vi "Build.vi"(6 "Assembly Type":string, 8 "Position":i32, 9 "XYZTheta":dbl[](array[numeric]), 10 "text file":dbl[][](array[numeric]), 11 "Sensor Dispense in":refnum<class "Sensor Dispense.lvclass">) -> (3 "Sensor Dispense out":refnum<class "Sensor Dispense.lvclass">)   [LabVIEW 2021, in "Sensor Dispense.lvclass"]
uses:
  Projects/Sensor Dispense.lvclass
  C:/Users/User/Documents/Jessica_Code/Jessica_code_08062024/Gantry-CMU/UCSB-Gantry-HEP-main/Classes/Routine/Dispense/Dispense.lvclass
  Projects/Sensor Dispense.lvclass/Sensor Dispense.ctl
  <vilib>/Analysis/coordinate.llb/2D Cartesian Coordinate Rotation (Scalar).vi
  <vilib>/Analysis/NI_AALPro.lvlib
panel:
  out "CW/CCW":dbl[](array[numeric])
  out "CW/CCW":dbl[](array[numeric])
  out "endpoints 2":dbl[][](array[numeric])
  out "endpoints":dbl[][](array[numeric])
  out "data":T1(array[cluster])
  out "cell count":dbl[](array[numeric])
  out "centers":dbl[][](array[numeric])
  # "[x1,y1,x2,y2]"
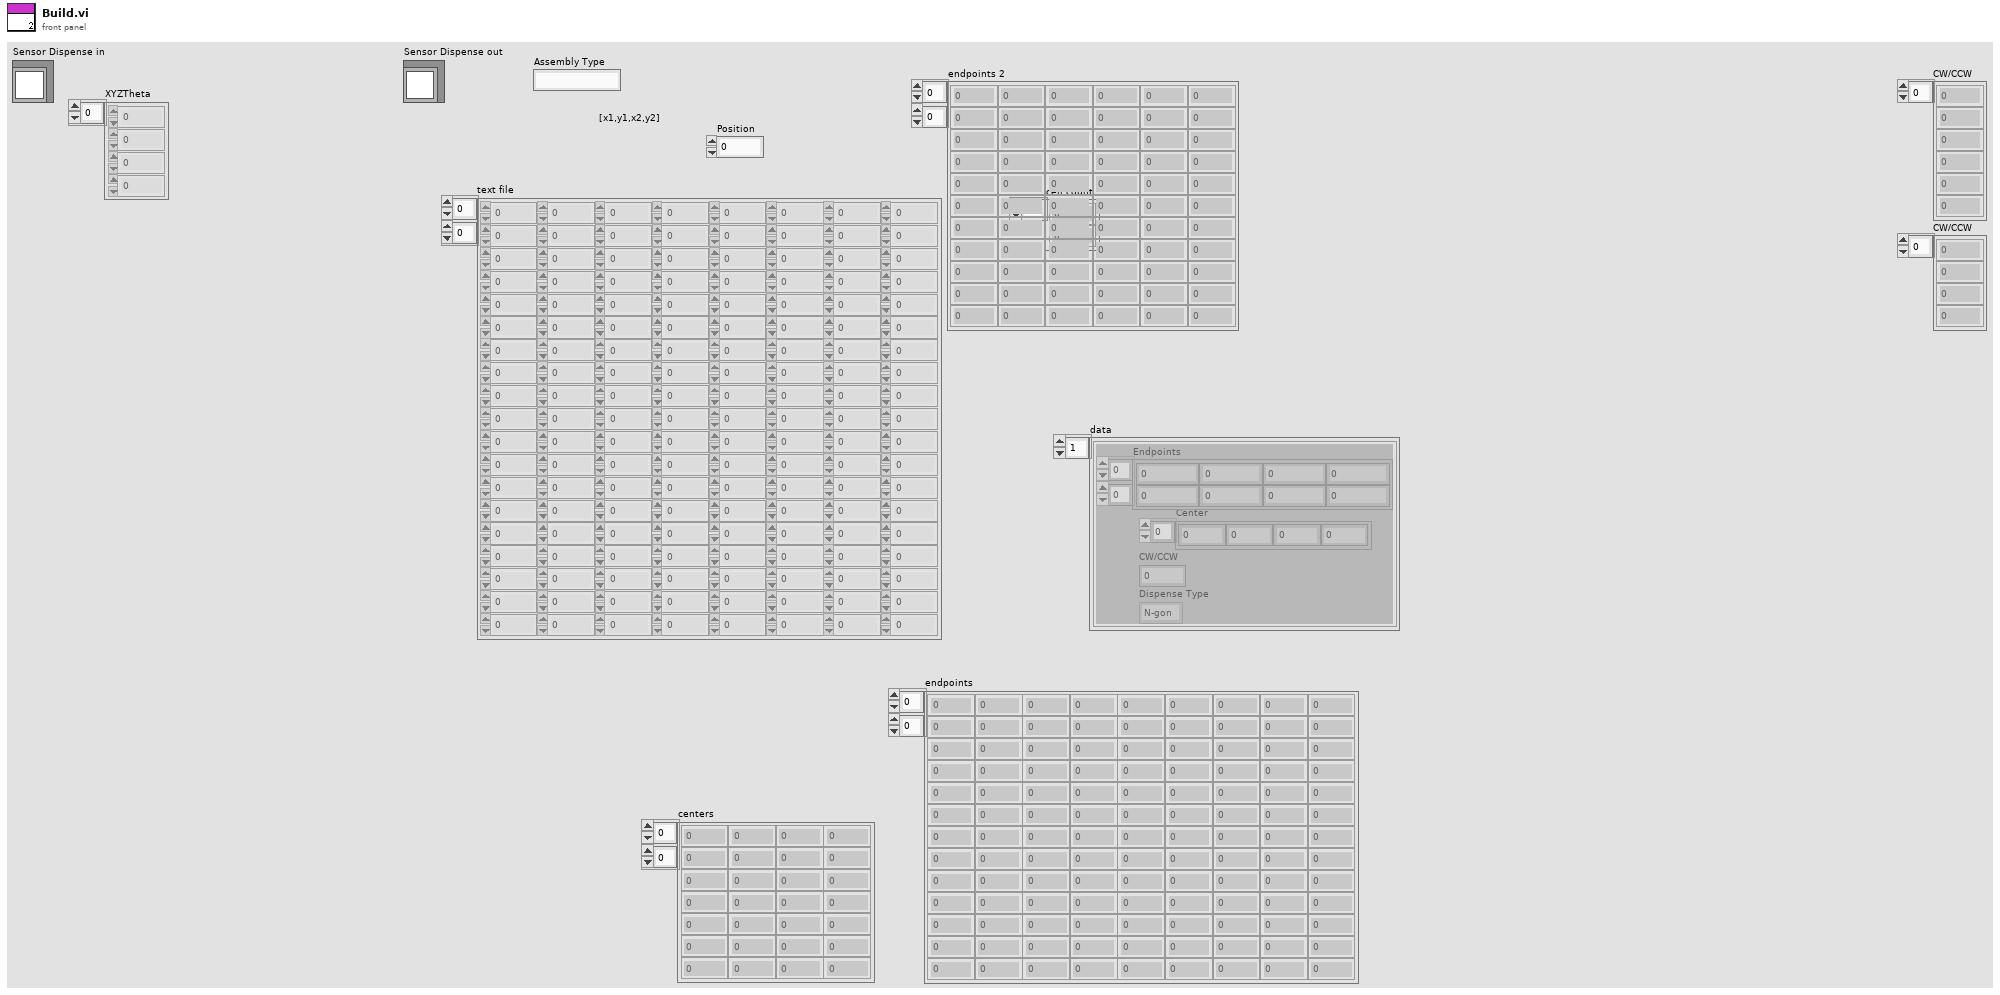
[diagram p1: front panel]
types:
  T1 = cluster{"Endpoints":dbl[][], "Center":dbl[], "CW/CCW":dbl, "Dispense Type":enum16{"N-gon", "Square", "Arc", "Dot", "Line", "Circle"}}[]
  T2 = enum16{"N-gon", "Square", "Arc", "Dot", "Line", "Circle"}
  T3 = cluster{"Endpoints":dbl[][], "Center":dbl[], "CW/CCW":dbl, "Dispense Type":enum16{"N-gon", "Square", "Arc", "Dot", "Line", "Circle"}}
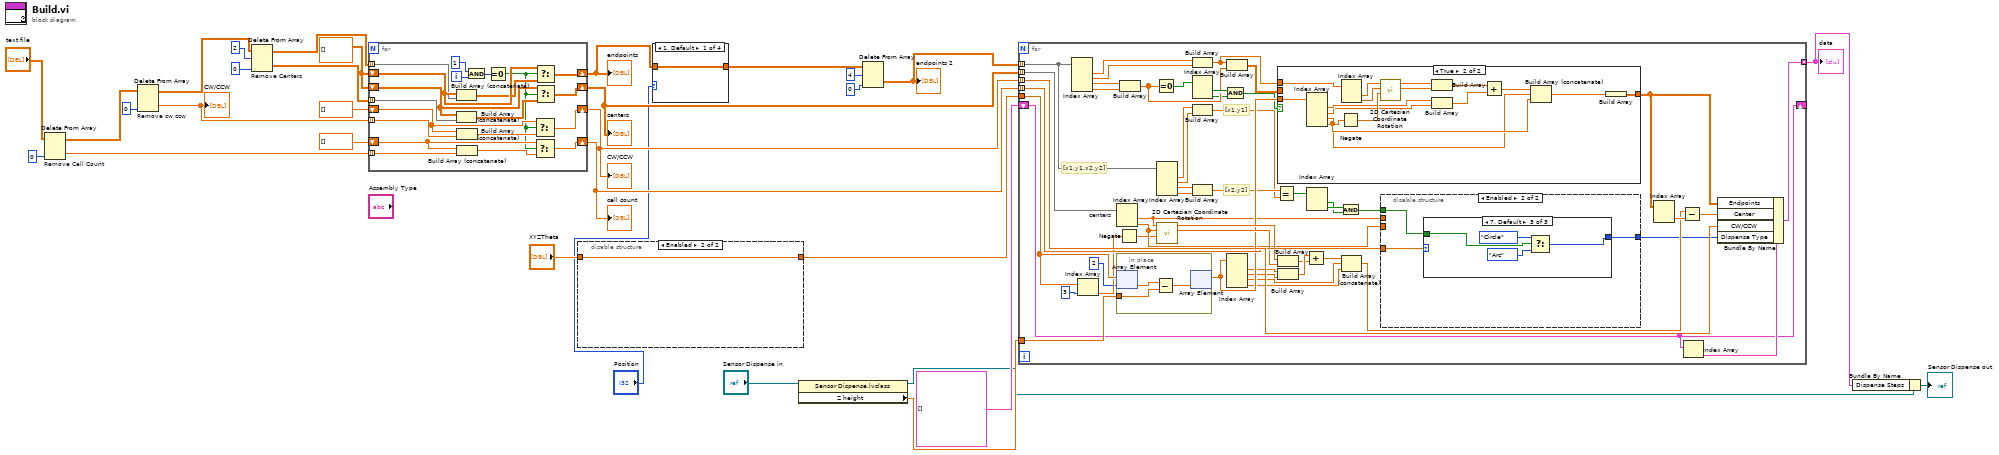
[diagram p0: block diagram]
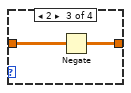
[diagram p3: hidden frame]
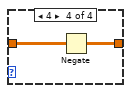
[diagram p4: hidden frame]
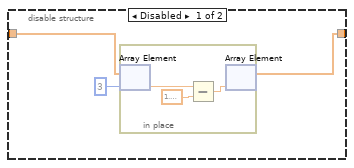
[diagram p5: hidden frame]
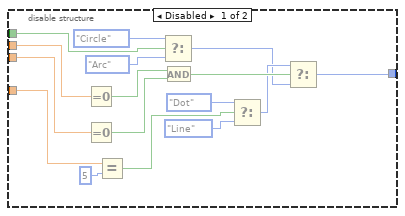
[diagram p6: hidden frame]
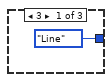
[diagram p7: hidden frame]
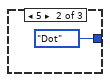
[diagram p8: hidden frame]
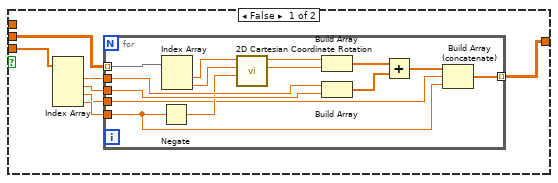
[diagram p9: hidden frame]
diagram:
  w28 = dbl[][] []
  n1 = Delete From Array "Remove Cell Count"(array="text file", index (col)=0) -> (deleted portion=w22:dbl[], array with subset deleted=w24:dbl[][])  [unwired: 2 in]
  n2 = Delete From Array "Remove cw ccw"(array=w24, index (col)=0 ("disabled index (col)")) -> (deleted portion=w5:dbl[], array with subset deleted=w21:dbl[][])  [unwired: 2 in]
  "CW/CCW" <- w5
  n3 = Delete From Array "Remove Centers"(array=w21, length=2, index (col)=0) -> (deleted portion=w17:dbl[][], array with subset deleted=w18:dbl[][])  [unwired: 1 in]
  n4 = for {
    tunnel: w18 -> [w47] mode=indexing
    shift-right: [w45] -> w1
    shift-left: w28 -> [w48]
    tunnel: w17 -> [w44] mode=indexing
    shift-right: [w41] -> w29
    shift-left: w28 -> [w42]
    tunnel: w22 -> [w40] mode=indexing
    shift-right: [w37] -> w26
    shift-left: dbl[] [] -> [w39]
    shift-right: [w32] -> w4
    shift-left: dbl[] [] -> [w35]
    tunnel: w5 -> [w36] mode=indexing
    i -> [w50]
    n5 = Build Array (concatenate)(w48, w47) -> (w46:dbl[][])
    n6 = Build Array (concatenate)(w42, w44) -> (w43:dbl[][])
    n7 = Build Array (concatenate)(w35, w36) -> (w34:dbl[])
    n8 = Build Array (concatenate)(w39, w40) -> (w38:dbl[])
    n9 = And(x=1, y=w50) -> (x .and. y?=w49:i32)
    n10 = Equal To 0?(x=w49) -> (x = 0?=w33:bool)
    n11 = Select(t=w35, s=w33, f=w34) -> (s? t:f=w32:dbl[])
    n12 = Select(t=w39, s=w33, f=w38) -> (s? t:f=w37:dbl[])
    n13 = Select(t=w48, s=w33, f=w46) -> (s? t:f=w45:dbl[][])
    n14 = Select(t=w42, s=w33, f=w43) -> (s? t:f=w41:dbl[][])
  }
  "centers" <- w29
  "cell count" <- w26
  "endpoints" <- w1
  "CW/CCW" <- w4
  n15 = disable-structure shown="Enabled" {
    disable-tunnel: "XYZTheta" -> [w54 w58]
    disable-tunnel: [w52 w58] -> w7
    frame Disabled {
      n16 = in-place {
        n17 = in-place-array #1(w54, 3) -> (w57:dbl)
        n18 = Subtract(x=w57, y=1.5707963267948966) -> (x-y=w55:dbl)
        n19 = in-place-array #1(w55) -> (w52:dbl[])  [unwired: 1 out]
      }
    }
    frame Enabled {
    }
  }
  n20 = case shown="1, Default" "Position" {
    tunnel: [w59 w60 w62 w64] -> w2
    tunnel: w1 -> [w59 w60 w61 w63]
    frame 1, Default {
    }
    frame 3 {
    }
    frame 2 {
      n21 = Negate(x=w61) -> (-x=w62:dbl[][])
    }
    frame 4 {
      n22 = Negate(x=w63) -> (-x=w64:dbl[][])
    }
  }
  n23 = property class="Sensor Dispense.lvclass"(reference="Sensor Dispense in") -> (reference out=w14:refnum<class "Sensor Dispense.lvclass">, "Z height"=w31:dbl)  [unwired: 1 in, 1 out]
  n24 = Delete From Array(array=w2, length=4, index (col)=0 ("disabled index (col)")) -> (deleted portion=w9:dbl[][])  [unwired: 1 in, 1 out]
  "endpoints 2" <- w9
  n25 = for {
    tunnel: w9 -> [w78] mode=indexing
    tunnel: w7 -> [w88]
    tunnel: w31 -> [w115]
    tunnel: w29 -> [w114] mode=indexing
    tunnel: w4 -> [w113] mode=indexing
    tunnel: w26 -> [w112] mode=indexing
    shift-right: [w97] -> _
    shift-left: T1 [] ("Dispense Steps") -> [w97]
    tunnel: [w111] -> w13 mode=indexing
    # "[x2,y2]"
    # "[x1,y1]"
    # "[x1,y1,x2,y2]"
    n26 = Index Array(array=w78) -> (element #1=w76:dbl, element #2=w75:dbl, element #3=w74:dbl, element #4=w73:dbl)  [unwired: 4 in]
    n27 = Index Array(array=w88, index=3) -> (element=w87:dbl)
    n28 = Index Array "centers"(array=w114) -> (element #1=w100:dbl, element #2=w99:dbl)  [unwired: 2 in]
    n29 = in-place {
      in-place-border: w115 -> [w142]
      n30 = in-place-array #2(w88, 2) -> (w143:dbl)
      n31 = Subtract(x=w143, y=w142) -> (x-y=w141:dbl)
      n32 = in-place-array #2(w141) -> (w108:dbl[])  [unwired: 1 out]
    }
    n33 = Negate(x=w87) -> (-x=w86:dbl)
    n34 = Build Array(w74, w73) -> (w70:dbl[])
    n35 = Equal To 0?(x=w70) -> (x = 0?=w69:bool[])
    n36 = Index Array(array=w78) -> (element #1=w84:dbl, element #2=w83:dbl, element #3=w96:dbl, element #4=w95:dbl)  [unwired: 4 in]
    n37 = call-poly <vilib>:"2D Cartesian Coordinate Rotation.vi"("theta"=w86, "y"=w99, "x"=w100) -> ("y out"=w109:dbl, "x out"=w110:dbl)  [unwired: 6 in, 1 out]
    n38 = Build Array(w76, w75) -> (w66:dbl[])
    n39 = Index Array(array=w69) -> (element #1=w71:bool, element #2=w67:bool)  [unwired: 2 in]
    n40 = Build Array(w84, w83) -> (w93:dbl[])
    n41 = Build Array(w96, w95) -> (w94:dbl[])
    n42 = And(x=w71, y=w67) -> (x .and. y?=w68:bool)
    n43 = Build Array(w66, w70) -> (w72:dbl[][])
    n44 = Index Array(array=w108) -> (element #1=w107:dbl, element #2=w104:dbl, element #3=w102:dbl, element #4=w101:dbl)  [unwired: 4 in]
    n45 = Equal?(x=w94, y=w93) -> (x = y?=w92:bool[])
    n46 = case shown="True" w68 {
      tunnel: w108 -> [w150 w177]
      tunnel: [w149 w165] -> w82
      tunnel: w72 -> [w148 _]
      tunnel: w66 -> [_ w180]
      frame False {
        n47 = Index Array(array=w150) -> (element #1=w147:dbl, element #2=w146:dbl, element #3=w144:dbl, element #4=w145:dbl)  [unwired: 4 in]
        n48 = for {
          tunnel: w148 -> [w164] mode=indexing
          tunnel: w147 -> [w161]
          tunnel: w146 -> [w160]
          tunnel: [w151] -> w149 mode=indexing
          tunnel: w145 -> [w152]
          tunnel: w144 -> [w153]
          n49 = Negate(x=w152) -> (-x=w155:dbl)
          n50 = Index Array(array=w164) -> (element #1=w163:dbl, element #2=w162:dbl)  [unwired: 2 in]
          n51 = call-poly <vilib>:"2D Cartesian Coordinate Rotation.vi"("theta"=w155, "y"=w162, "x"=w163) -> ("y out"=w158:dbl, "x out"=w159:dbl)  [unwired: 6 in, 1 out]
          n52 = Build Array(w159, w158) -> (w157:dbl[])
          n53 = Build Array(w161, w160) -> (w156:dbl[])
          n54 = Add(x=w157, y=w156) -> (x+y=w154:dbl[])
          n55 = Build Array (concatenate)(w154, w153, w152) -> (w151:dbl[])
        }
      }
      frame True {
        n56 = Index Array(array=w177) -> (element #1=w173:dbl, element #2=w172:dbl, element #3=w168:dbl, element #4=w169:dbl)  [unwired: 4 in]
        n57 = Negate(x=w169) -> (-x=w176:dbl)
        n58 = Index Array(array=w180) -> (element #1=w179:dbl, element #2=w178:dbl)  [unwired: 2 in]
        n59 = call-poly <vilib>:"2D Cartesian Coordinate Rotation.vi"("theta"=w176, "y"=w178, "x"=w179) -> ("y out"=w174:dbl, "x out"=w175:dbl)  [unwired: 6 in, 1 out]
        n60 = Build Array(w175, w174) -> (w170:dbl[])
        n61 = Build Array(w173, w172) -> (w171:dbl[])
        n62 = Add(x=w170, y=w171) -> (x+y=w167:dbl[])
        n63 = Build Array (concatenate)(w167, w168, w169) -> (w166:dbl[])
        n64 = Build Array(w166) -> (w165:dbl[][])
      }
    }
    n65 = Build Array(w110, w109) -> (w105:dbl[])
    n66 = Build Array(w107, w104) -> (w106:dbl[])
    n67 = Add(x=w106, y=w105) -> (x+y=w103:dbl[])
    n68 = Index Array(array=w92) -> (element #1=w90:bool, element #2=w91:bool)  [unwired: 2 in]
    n69 = And(x=w91, y=w90) -> (x .and. y?=w89:bool)
    n70 = Build Array (concatenate)(w103, w102, w101) -> (w80:dbl[])
    n71 = disable-structure shown="Enabled" {
      disable-tunnel: w112 -> [w131 w134]
      disable-tunnel: w100 -> [w128 _]
      disable-tunnel: w99 -> [w127 _]
      disable-tunnel: w89 -> [w120 w133]
      disable-tunnel: [w116 w132] -> w77
      frame Disabled {
        n72 = Equal To 0?(x=w128) -> (x = 0?=w129:bool)
        n73 = Equal To 0?(x=w127) -> (x = 0?=w130:bool)
        n74 = Equal?(x=w131, y=5) -> (x = y?=w123:bool)
        n75 = Select(t=T2."Circle" ("Dispense Type"), s=w120, f=T2."Arc" ("Dispense Type")) -> (s? t:f=w117:T2)
        n76 = And(x=w129, y=w130) -> (x .and. y?=w119:bool)
        n77 = Select(t=T2."Dot" ("Dispense Type"), s=w123, f=T2."Line" ("Dispense Type")) -> (s? t:f=w118:T2)
        n78 = Select(t=w118, s=w119, f=w117) -> (s? t:f=w116:T2)
      }
      frame Enabled {
        n79 = case shown="7, Default" w134 {
          tunnel: w133 -> [_ _ w138]
          tunnel: [T2."Line" ("Dispense Type") T2."Dot" ("Dispense Type") w137] -> w132
          frame 3 {
          }
          frame 5 {
          }
          frame 7, Default {
            n80 = Select(t=T2."Circle" ("Dispense Type"), s=w138, f=T2."Arc" ("Dispense Type")) -> (s? t:f=w137:T2)
          }
        }
      }
    }
    n81 = Index Array(array=w82) -> (element=w81:dbl[])  [unwired: 2 in]
    n82 = Subtract(x=w80, y=w81) -> (x-y=w79:dbl[])
    n83 = Index Array(array=w97) -> (element=w98:T3)  [unwired: 1 in]
    n84 = Bundle By Name(cluster=w98, "Endpoints"=w82, "Center"=w79, "CW/CCW"=w113, "Dispense Type"=w77) -> (w111:T3)
  }
  "data" <- w13
  n85 = Bundle By Name(cluster=w14, "Dispense Steps"=w13) -> (→"Sensor Dispense out":refnum<class "Sensor Dispense.lvclass">)
